vi "porog.vi"(1 "Array":i16[](array[numeric])) -> (0 "Numeric":dbl)   [LabVIEW 2010]
uses:
  <vilib>/Analysis/NI_AALBase.lvlib
panel:
  out "Histogram Graph":T1(graph)
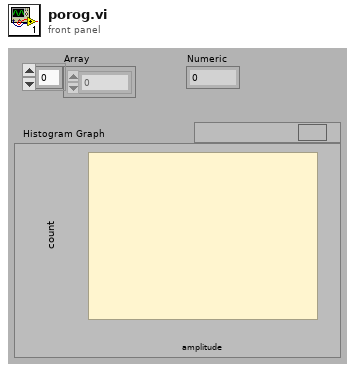
[diagram p1: front panel]
types:
  T1 = cluster{"X Values":dbl[], "Histogram: h(x)":i32[]}
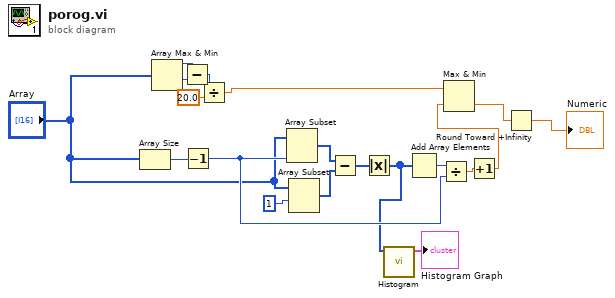
[diagram p0: block diagram]
diagram:
  n1 = Array Size(array="Array") -> (size(s)=w10:i32)
  n2 = Array Max & Min(array="Array") -> (max value=w4:i16, min value=w5:i16)  [unwired: 2 out]
  n3 = Subtract(x=w4, y=w5) -> (x-y=w7:i16)
  n4 = Decrement(x=w10) -> (x-1=w14:i32)
  n5 = Divide(x=w7, y=20.0) -> (x/y=w16:dbl)
  n6 = Array Subset(array="Array", length=w14) -> (w11:i16[])  [unwired: 1 in]
  n7 = Array Subset(array="Array", index=1) -> (w12:i16[])  [unwired: 1 in]
  n8 = Subtract(x=w11, y=w12) -> (x-y=w3:i16[])
  n9 = Absolute Value(x=w3) -> (abs(x)=w1:i16[])
  n10 = call <vilib>:"Histogram.vi"("X"=w1) -> ("Histogram Graph"=→"Histogram Graph":T1)  [unwired: 7 in, 3 out]
  n11 = Add Array Elements(numeric array=w1) -> (sum=w13:i16)
  n12 = Divide(x=w13, y=w14) -> (x/y=w15:dbl)
  n13 = Increment(x=w15) -> (x+1=w17:dbl)
  n14 = Max & Min(x=w16, y=w17) -> (min(x,y)=w18:dbl)  [unwired: 1 out]
  n15 = Round Toward +Infinity(x=w18) -> (ceil(x): smallest int >= x=→"Numeric":dbl)
